vi "Mod_OFDM_Examine_Configure_Pulse_Shaping_Parameters.vi"(0 "Configuration in":variant, 11 "error in":errorcluster) -> (4 "Configuration out":variant, 15 "error out":errorcluster)   [LabVIEW 2010]
doc: "The VI allows the user to examine/configure the pulse shaping parameters that is used for upsampling during waveform generation. Following parameters are configured.\n\nSamples per Symbol: Specifies the number of desired samples per symbol for the pulse shaping filter. Specify an even number >2. \n\nTX Filter: Specifies the class of filter to generate. Following three options are available:\n1. None\n2. Raised Cosine\n3. Root Raised Cosine\n\nAlpha: This is a filter parameter which specifies the rolloff for raised cosine and square root raised cosine filters. This input is ignored when the TX filter is set to none. \n\nFilter Length: Specifies the desired length of the pulse shaping filter, measured in symbols. The length of the matched filter can vary according to filter type and modulation type. Valid values are > 1. \n\nSymbol rate: specifies the desired symbol rate in units of Hz."
uses:
  Polymorphic_Sub_VI's/Mod_OFDM_Get_Pulse_Shaping.vi
  Polymorphic_Sub_VI's/Mod_OFDM_Set_Pulse_Shaping_Parameters.vi
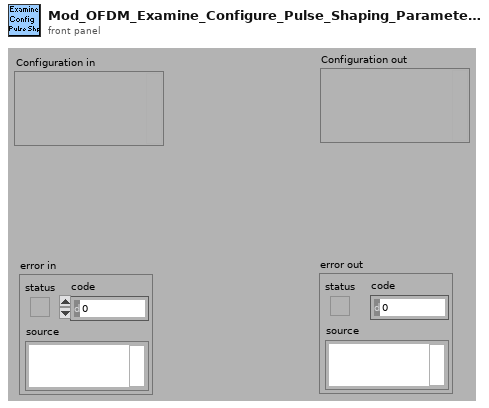
[diagram p1: front panel]
types:
  T1 = typedef "Configure Pulse Shaping.ctl" = cluster{"System Filter":cluster{"TX Filter":enum16{"none", "Raised Cosine", "Root Raised Cos"}, "Alpha":dbl, "filter length":i32}, "Modulation system parameters":cluster{"samples per symbol (16)":u32}, "symbol rate (Hz)":dbl}
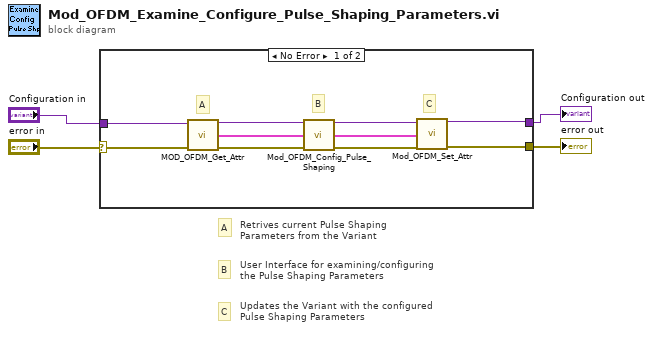
[diagram p0: block diagram]
diagram:
  # "Updates the Variant with the configured Pulse Shaping Parameters"
  # "User Interface for examining/configuring the Pulse Shaping Parameters"
  # "Retrives current Pulse Shaping Parameters from the Variant"
  # "A"
  # "C"
  # "B"
  n1 = case shown="No Error" "error in" {
    selector: "error in" -> [w5 w15]
    tunnel: "Configuration in" -> [w12 _]
    tunnel: [w11 w15] -> w3
    tunnel: [w10 _] -> w2
    frame No Error {
      # "C"
      # "B"
      # "A"
      n2 = call-poly "MOD_OFDM_Get_Attr.vi"("Configuration in"=w12, "error in"=w5) -> ("Configuration out"=w9:variant, "Pulse Shaping"=w7:T1, "error out"=w13:errorcluster)  [unwired: 10 in, 1 out]
      n3 = call "Mod_OFDM_Config_Pulse_Shaping.vi"("Configuration in"=w9, "Pulse Shaping"=w7, "error in"=w13) -> ("Configuration out"=w8:variant, "Pulse Shaping"=w6:T1, "error out"=w14:errorcluster)  [unwired: 10 in]
      n4 = call-poly "Mod_OFDM_Set_Attr.vi"("Configuration in"=w8, "Pulse Shaping"=w6, "error in"=w14) -> ("Configuration out"=w10:variant, "error out"=w11:errorcluster)  [unwired: 11 in]
    }
    frame Error {
    }
  }
  "error out" <- w3
  "Configuration out" <- w2
